vi "BCtr_1_Init.vi"(8 "error in (no error)":errorcluster, 11 "SBPort":string) -> (0 "error out":errorcluster, 3 "CtrCfg":T1 {"BaseAddrOut" format="%x"})   [LabVIEW 2016]
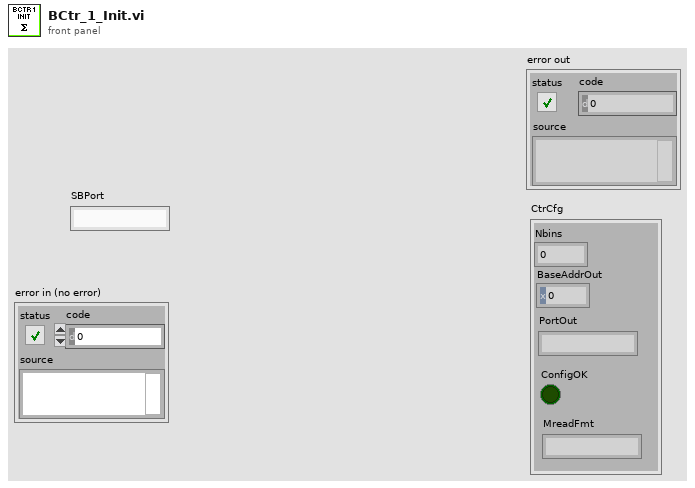
[diagram p1: front panel]
types:
  T1 = cluster{"Nbins":u16, "BaseAddrOut":u16, "PortOut":string, "ConfigOK":bool, "MreadFmt":string}
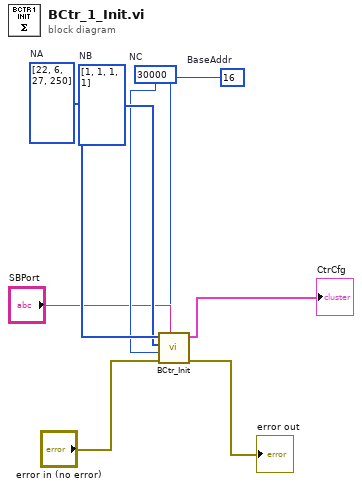
[diagram p0: block diagram]
diagram:
  w2 = u16 16  # BaseAddr
  w6 = u32 30000  # NC
  w7 = u16[] [1, 1, 1, 1]  # NB
  w8 = u16[] [22, 6, 27, 250]  # NA
  n1 = call "BCtr_Init.vi"("BaseAddr"=w2, "SBPort"="SBPort", "error in (no error)"="error in (no error)", "NC"=w6, "NB"=w7, "NA"=w8) -> ("error out"=→"error out":errorcluster, "CtrCfg"=→"CtrCfg":T1)  [unwired: 4 in]
